vi "Is Initialized.vi"(8 "error in":errorcluster, 11 "Virtual NEO480 in":refnum<class "Virtual NEO480.lvclass">) -> (0 "error out":errorcluster, 2 "Is Initialized?":bool, 3 "Virtual NEO480 out":refnum<class "Virtual NEO480.lvclass">)   [LabVIEW 2024, in "Virtual NEO480.lvclass"]
uses:
  Virtual NEO480.lvclass
  Virtual NEO480.lvclass/Virtual NEO480.ctl
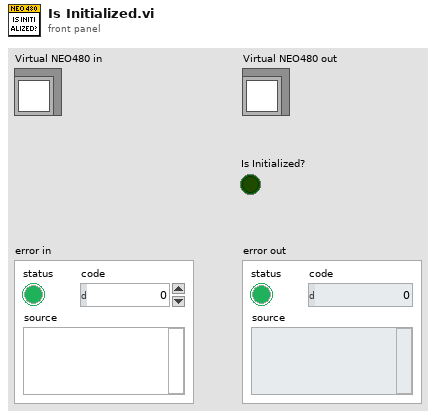
[diagram p1: front panel]
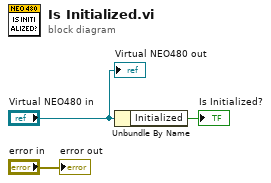
[diagram p0: block diagram]
diagram:
  n1 = Unbundle By Name("Virtual NEO480 in") -> ("Initialized"=→"Is Initialized?":bool)
  "Virtual NEO480 out" <- "Virtual NEO480 in"
  "error out" <- "error in"
